vi "xmltddresult for Q8X.vi"(9 "second result":string, 10 "TDD spec":string, 11 "TDD array":string[][](array[string])) -> (1 "pointValue":string[][](array[string]), 2 "TDD third result":string[][](array[string]))   [LabVIEW 2011]
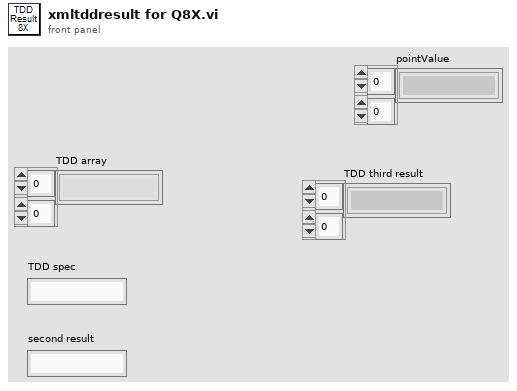
[diagram p1: front panel]
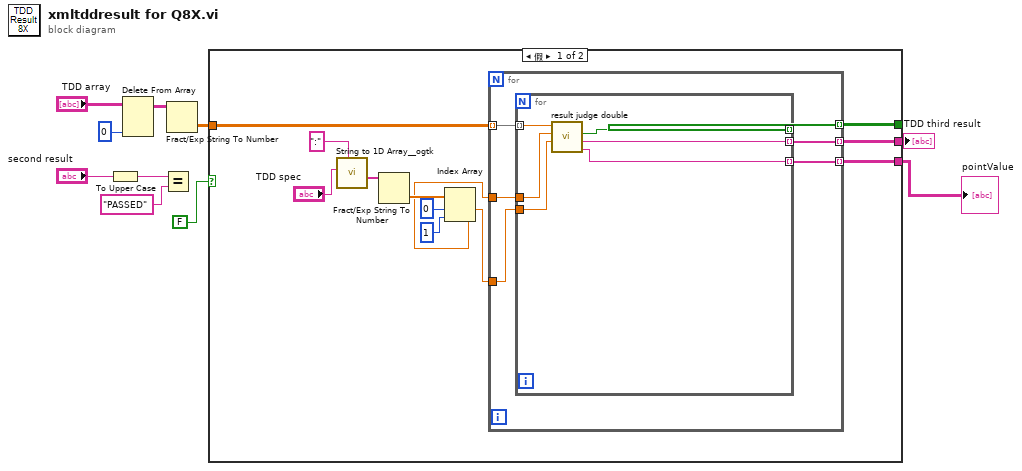
[diagram p0: block diagram]
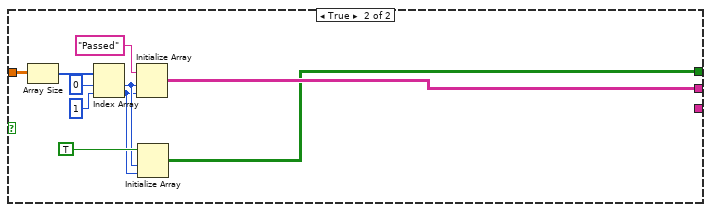
[diagram p2: hidden frame]
diagram:
  n1 = To Upper Case(1:"second result") -> (0:w5:string)
  n2 = Delete From Array(array="TDD array", index (col)=0 ("禁用的索引 (列)")) -> (array with subset deleted=w8:string[][])  [unwired: 2 in, 1 out]
  n3 = Equal?(x=w5, y="PASSED") -> ()  [unwired: 1 out]
  n4 = Fract/Exp String To Number(string=w8) -> (number=w7:dbl[][])  [unwired: 3 in, 1 out]
  n5 = case shown="假" FALSE {
    tunnel: w7 -> [w19 w44]
    tunnel: [w13 w39] -> w3
    tunnel: [w12 w35] -> _
    tunnel: [w11 _] -> w2
    frame False {
      n6 = call <userlib>:"String to 1D Array__ogtk.vi"("delimiter (Tab)"=":", "string"="TDD spec") -> ("Array of Strings"=w20:string[])  [unwired: 9 in]
      n7 = Fract/Exp String To Number(string=w20) -> (number=w16:dbl[])  [unwired: 3 in, 1 out]
      n8 = Index Array(array=w16, index #1=0 ("索引"), index #2=1 ("索引")) -> (element #1=w15:dbl, element #2=w14:dbl)
      n9 = for {
        tunnel: w19 -> [w28] mode=indexing
        tunnel: w15 -> [w27]
        tunnel: w14 -> [w26]
        tunnel: [w25] -> w13 mode=indexing
        tunnel: [w24] -> w12 mode=indexing
        tunnel: [w23] -> w11 mode=indexing
        n10 = for {
          tunnel: w28 -> [w34] mode=indexing
          tunnel: w27 -> [w33]
          tunnel: w26 -> [w32]
          tunnel: [w31] -> w25 mode=indexing
          tunnel: [w30] -> w24 mode=indexing
          tunnel: [w29] -> w23 mode=indexing
          n11 = call "result judge double.vi"("lower limit"=w33, "upper limit"=w32, "test value"=w34) -> ("pointValue"=w29:string, "result string"=w31:string, "result"=w30:bool)  [unwired: 6 in]
        }
      }
    }
    frame True {
      n12 = Array Size(array=w44) -> (size(s)=w43:i32[])
      n13 = Index Array(array=w43, index #1=0 ("索引"), index #2=1 ("索引")) -> (element #1=w37:i32, element #2=w36:i32)
      n14 = Initialize Array("Passed" ("TrueValue"), w37, w36) -> (w39:string[][])
      n15 = Initialize Array(TRUE, w37, w36) -> (w35:bool[][])
    }
  }
  "TDD third result" <- w3
  "pointValue" <- w2
